vi "5.for-loop.vi"() -> ()   [LabVIEW 2010]
panel:
  in  "# of time to  run":dbl
  out "current-iteration-no":dbl
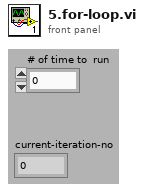
[diagram p1: front panel]
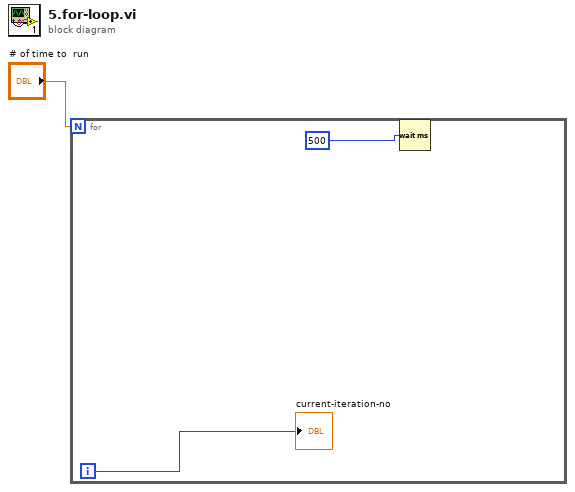
[diagram p0: block diagram]
diagram:
  n1 = for {
    N: "# of time to  run" -> [_]
    i -> [w3]
    n2 = Wait (ms)(milliseconds to wait=500) -> ()  [unwired: 1 out]
    "current-iteration-no" <- w3
  }
